vi "LogTimeDataExtract.vi"() -> ()   [LabVIEW 2014]
uses:
  ColumnData.ctl
  <vilib>/Analysis/NI_AALBase.lvlib
panel:
  out "Busy Interval Histogram":T1(graph)
  out "Busy Delay Histogram":T1(graph)
  out "Audible Read Interval Mean":dbl format="%0.4f"
  out "Audible Read Interval Histogram":T1(graph)
  out "Audible Read Start Delay Histogram":T1(graph)
  out "Column Repeat Sample Size":i32
  out "Column Switch Sample Size":i32
  out "Audible Read Start Delay Mean":dbl format="%0.4f"
  out "Column Repeat Command Delay Histogram":T1(graph)
  out "Column Switch Command Delay Histogram":T1(graph)
  out "Column Switch Command Delay Mean":dbl format="%0.4f"
  out "Column Repeat Command Delay Mean":dbl format="%0.4f"
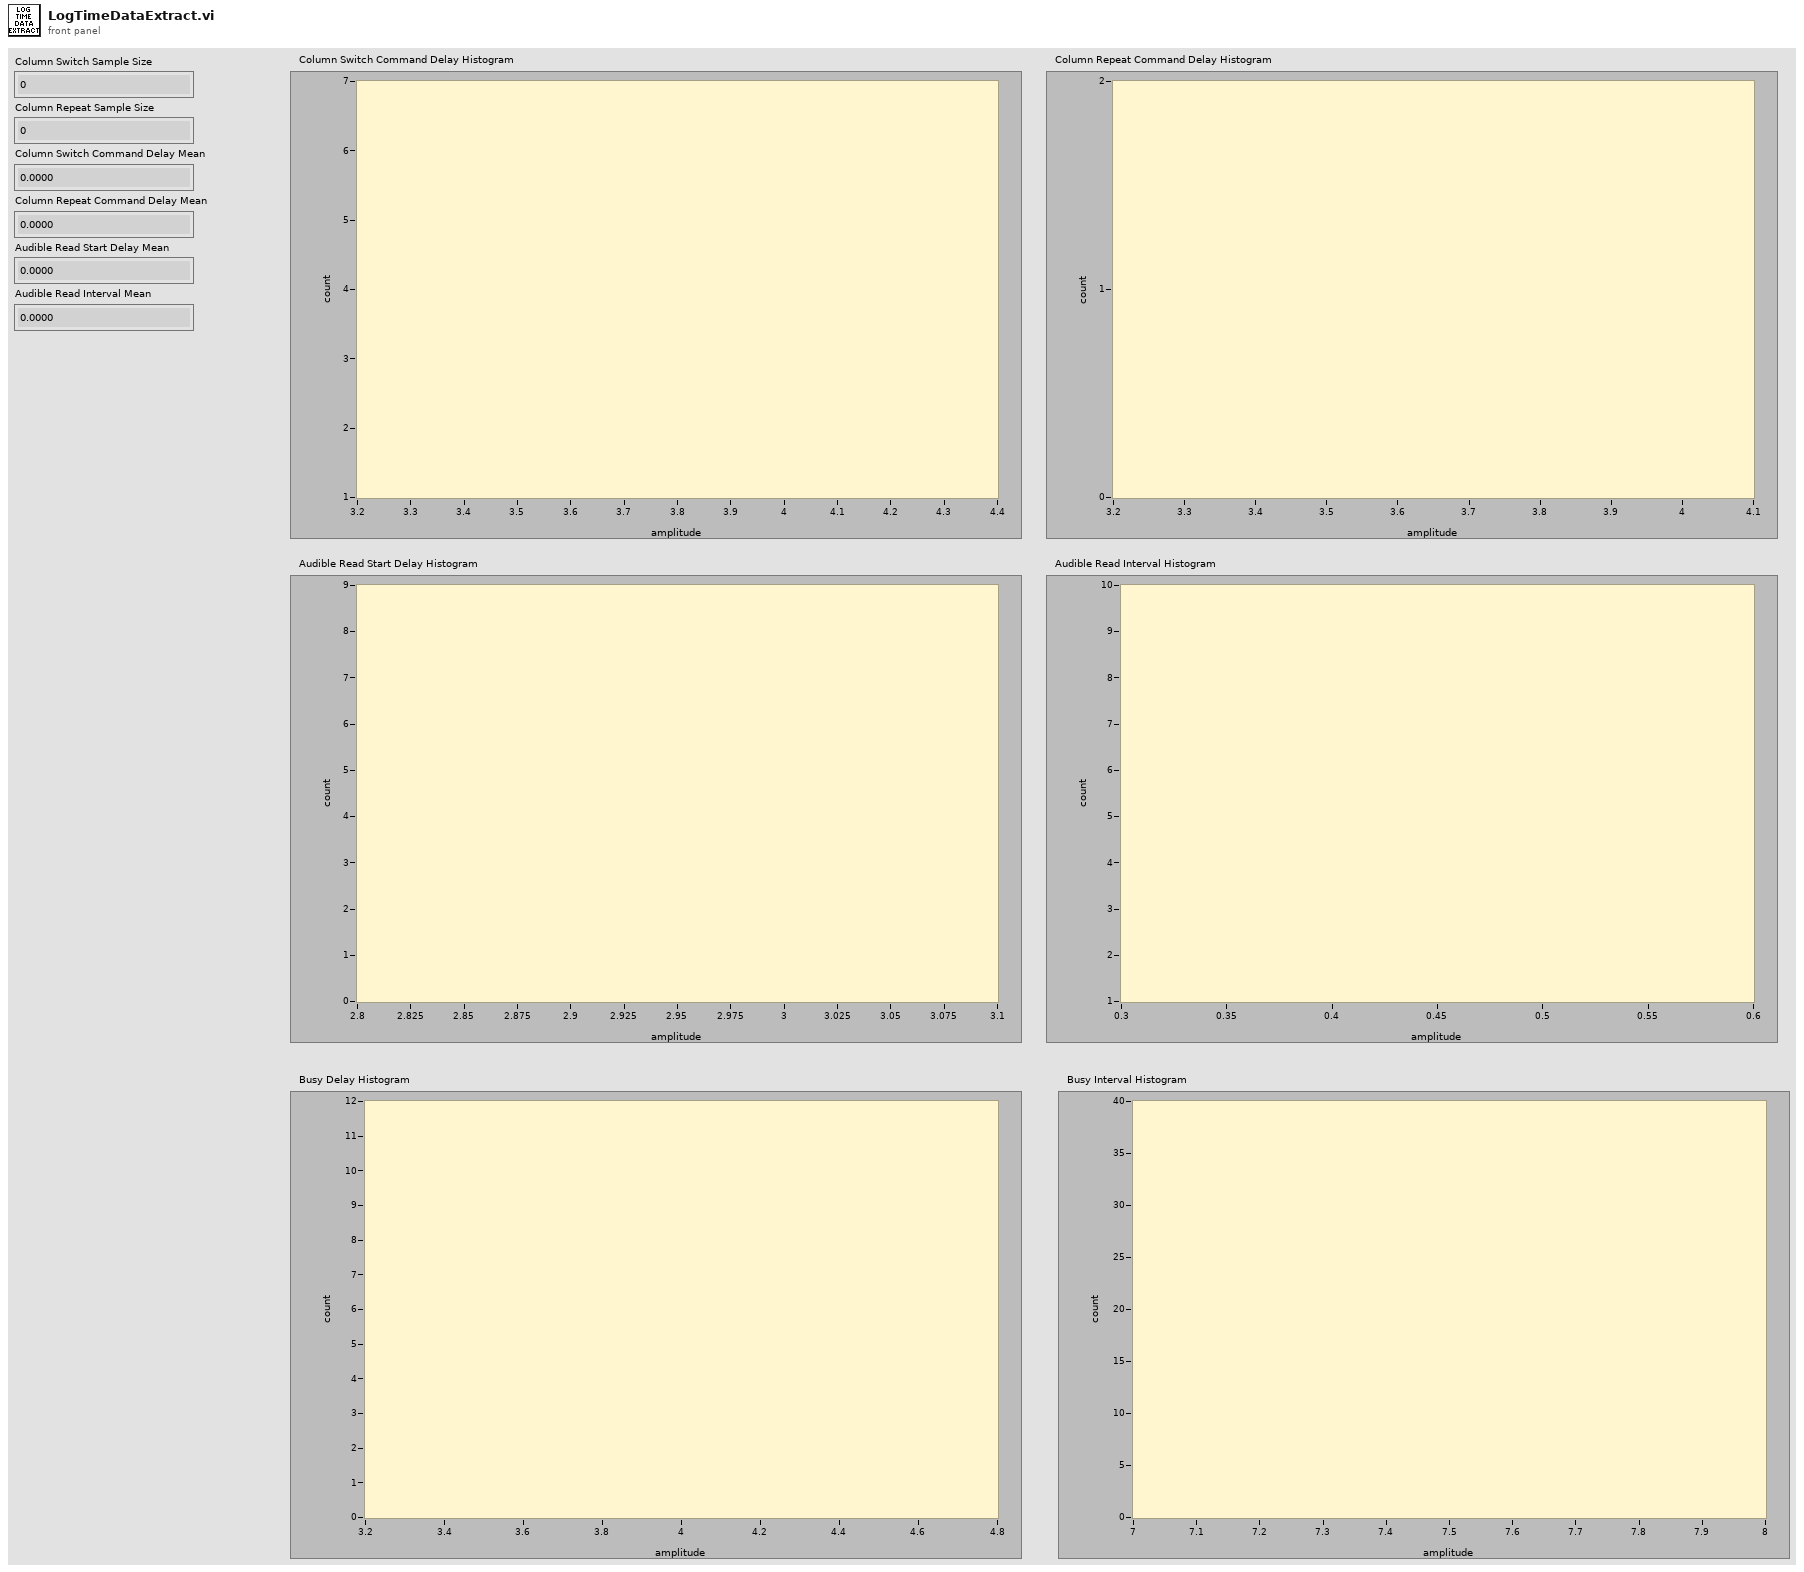
[diagram p1: front panel]
types:
  T1 = cluster{"X Values":dbl[], "Histogram: h(x)":i32[]}
  T2 = typedef "ColumnData.ctl" = cluster{"Col Absorbances":dbl[], "Col Read Times":timestamp[], "Col Read Positions (deg)":dbl[], "Temperature (degC)":dbl, "Active Column":u64, "Previous Column":u64, "Column Read Start Time":timestamp, "Column Busy Start Time":timestamp, "Column Busy Stop Time":timestamp, "Column Mark Read Start Time":timestamp, "Column Mark Read Stop Time":timestamp}
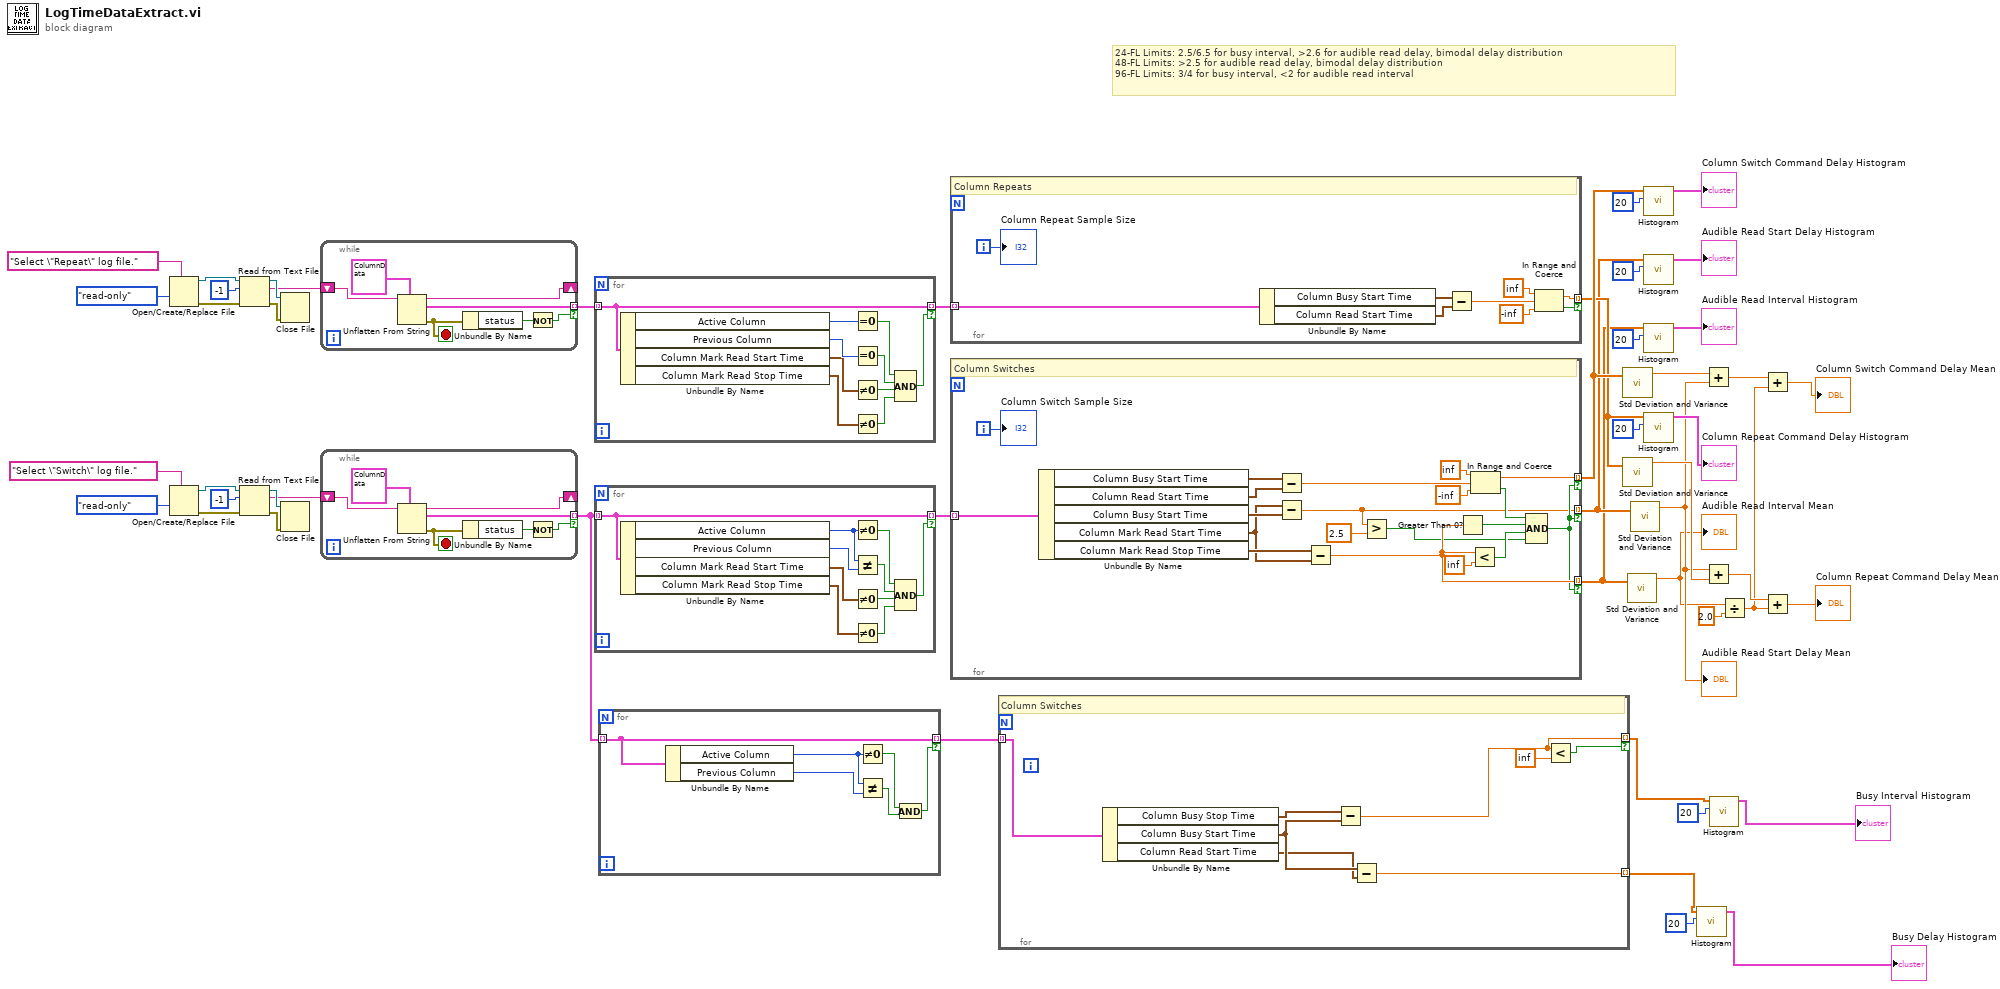
[diagram p0: block diagram]
diagram:
  # "24-FL Limits: 2.5/6.5 for busy interval, >2.6 for audible read delay, bimodal delay distribution\n48-FL Limits: >2.5 for audible read delay, bimodal delay distribution\n96-FL Limits: 3/4 for busy interval, <2 for audible read interval"
  n1 = Open/Create/Replace File(prompt="Select \"Repeat\" log file.", access (0:read/write)=enum16{"read/write", "read-only", "write-only"}."read-only") -> (refnum out=w38:refnum<file>, error out=w35:errorcluster)  [unwired: 4 in, 1 out]
  n2 = Open/Create/Replace File(prompt="Select \"Switch\" log file.", access (0:read/write)=enum16{"read/write", "read-only", "write-only"}."read-only") -> (refnum out=w49:refnum<file>, error out=w46:errorcluster)  [unwired: 4 in, 1 out]
  n3 = Read from Text File(file (use dialog)=w38, count=-1, error in=w35) -> (refnum out=w36:refnum<file>, text=w31:string, error out=w34:errorcluster)  [unwired: 1 in, 1 out]
  n4 = Read from Text File(file (use dialog)=w49, count=-1, error in=w46) -> (refnum out=w47:refnum<file>, text=w30:string, error out=w45:errorcluster)  [unwired: 1 in, 1 out]
  n5 = Close File(refnum=w36, error in=w34) -> ()  [unwired: 2 out]
  n6 = Close File(refnum=w47, error in=w45) -> ()  [unwired: 2 out]
  n7 = while {
    shift-right: [w55] -> _
    shift-left: w31 -> [w56]
    tunnel: [w54] -> w27 mode=indexing if=w50
    stop <- w52 stop-if-true
    n8 = Unflatten From String(type=T2 {"Col Absorbances"=[], "Col Read Times"=[], "Col Read Positions (deg)"=[], "Temperature (degC)"=0.0, "Active Column"=0, "Previous Column"=0, "Column Read Start Time"=timestamp(0 s since 1904-01-01), "Column Busy Start Time"=timestamp(0 s since 1904-01-01), "Column Busy Stop Time"=timestamp(0 s since 1904-01-01), "Column Mark Read Start Time"=timestamp(0 s since 1904-01-01), "Column Mark Read Stop Time"=timestamp(0 s since 1904-01-01)} ("Column Data"), binary string=w56) -> (rest of the binary string=w55:string, value=w54:T2, error out=w52:errorcluster)  [unwired: 3 in]
    n9 = Unbundle By Name(w52) -> ("status"=w51:bool)
    n10 = Not(x=w51) -> (.not. x?=w50:bool)
  }
  n11 = while {
    shift-right: [w62] -> _
    shift-left: w30 -> [w63]
    tunnel: [w61] -> w8 mode=indexing if=w57
    stop <- w59 stop-if-true
    n12 = Unflatten From String(type=T2 {"Col Absorbances"=[], "Col Read Times"=[], "Col Read Positions (deg)"=[], "Temperature (degC)"=0.0, "Active Column"=0, "Previous Column"=0, "Column Read Start Time"=timestamp(0 s since 1904-01-01), "Column Busy Start Time"=timestamp(0 s since 1904-01-01), "Column Busy Stop Time"=timestamp(0 s since 1904-01-01), "Column Mark Read Start Time"=timestamp(0 s since 1904-01-01), "Column Mark Read Stop Time"=timestamp(0 s since 1904-01-01)} ("Column Data"), binary string=w63) -> (rest of the binary string=w62:string, value=w61:T2, error out=w59:errorcluster)  [unwired: 3 in]
    n13 = Unbundle By Name(w59) -> ("status"=w58:bool)
    n14 = Not(x=w58) -> (.not. x?=w57:bool)
  }
  n15 = for {
    tunnel: w27 -> [w69] mode=indexing
    tunnel: [w69] -> w26 mode=indexing if=w68
    n16 = Unbundle By Name(w69) -> ("Active Column"=w73:u64, "Previous Column"=w72:u64, "Column Mark Read Start Time"=w67:timestamp, "Column Mark Read Stop Time"=w64:timestamp)
    n17 = Equal To 0?(x=w73) -> (x = 0?=w70:bool)
    n18 = Equal To 0?(x=w72) -> (x = 0?=w71:bool)
    n19 = Not Equal To 0?(x=w67) -> (x != 0?=w66:bool)
    n20 = Not Equal To 0?(x=w64) -> (x != 0?=w65:bool)
    n21 = Compound Arithmetic op=AND(w70, w71, w66, w65) -> (w68:bool)
  }
  n22 = for {
    tunnel: w8 -> [w83] mode=indexing
    tunnel: [w83] -> w9 mode=indexing if=w78
    n23 = Unbundle By Name(w83) -> ("Active Column"=w82:u64, "Previous Column"=w81:u64, "Column Mark Read Start Time"=w77:timestamp, "Column Mark Read Stop Time"=w75:timestamp)
    n24 = Not Equal To 0?(x=w82) -> (x != 0?=w80:bool)
    n25 = Not Equal?(x=w82, y=w81) -> (x != y?=w79:bool)
    n26 = Not Equal To 0?(x=w77) -> (x != 0?=w76:bool)
    n27 = Not Equal To 0?(x=w75) -> (x != 0?=w74:bool)
    n28 = Compound Arithmetic op=AND(w80, w79, w76, w74) -> (w78:bool)
  }
  n29 = for {
    tunnel: w8 -> [w89] mode=indexing
    tunnel: [w89] -> w7 mode=indexing if=w84
    n30 = Unbundle By Name(w89) -> ("Active Column"=w88:u64, "Previous Column"=w87:u64)
    n31 = Not Equal To 0?(x=w88) -> (x != 0?=w86:bool)
    n32 = Not Equal?(x=w88, y=w87) -> (x != y?=w85:bool)
    n33 = Compound Arithmetic op=AND(w86, w85) -> (w84:bool)
  }
  n34 = for {
    tunnel: w26 -> [w98] mode=indexing
    tunnel: [w93] -> w32 mode=indexing if=w92
    i -> [w95]
    # "Column Repeats"
    n35 = Unbundle By Name(w98) -> ("Column Busy Start Time"=w97:timestamp, "Column Read Start Time"=w96:timestamp)
    n36 = Subtract(x=w97, y=w96) -> (x-y=w94:dbl)
    n37 = In Range and Coerce(upper limit=inf, x=w94, lower limit=-inf) -> (coerced(x)=w93:dbl, In Range?=w92:bool)
    "Column Repeat Sample Size" <- w95
  }
  n38 = for {
    tunnel: w9 -> [w118] mode=indexing
    tunnel: [w115] -> w39 mode=indexing if=w104
    tunnel: [w103] -> w23 mode=indexing if=w104
    tunnel: [w112] -> w21 mode=indexing if=w104
    i -> [w116]
    # "Column Switches"
    n39 = Unbundle By Name(w118) -> ("Column Busy Start Time"=w117:timestamp, "Column Read Start Time"=w108:timestamp, "Column Busy Start Time"=w107:timestamp, "Column Mark Read Start Time"=w105:timestamp, "Column Mark Read Stop Time"=w106:timestamp)
    n40 = Subtract(x=w117, y=w108) -> (x-y=w109:dbl)
    n41 = Subtract(x=w105, y=w107) -> (x-y=w103:dbl)
    n42 = Subtract(x=w106, y=w105) -> (x-y=w112:dbl)
    n43 = Greater?(x=w103, y=2.5) -> (0:w102:bool)
    n44 = Greater Than 0?(x=w112) -> (x > 0?=w113:bool)
    n45 = Less?(x=w112, y=inf) -> (x < y?=w110:bool)
    n46 = In Range and Coerce(upper limit=inf, x=w109, lower limit=-inf) -> (coerced(x)=w115:dbl, In Range?=w114:bool)
    n47 = Compound Arithmetic op=AND(w114, w113, w110, w102) -> (w104:bool)
    "Column Switch Sample Size" <- w116
  }
  n48 = for {
    tunnel: w7 -> [w126] mode=indexing
    tunnel: [w122] -> w4 mode=indexing
    tunnel: [w120] -> w1 mode=indexing if=w119
    # "Column Switches"
    n49 = Unbundle By Name(w126) -> ("Column Busy Stop Time"=w125:timestamp, "Column Busy Start Time"=w124:timestamp, "Column Read Start Time"=w123:timestamp)
    n50 = Subtract(x=w125, y=w124) -> (x-y=w120:dbl)
    n51 = Subtract(x=w124, y=w123) -> (x-y=w122:dbl)
    n52 = Less?(x=w120, y=inf) -> (x < y?=w119:bool)
  }
  n53 = call <vilib>:"Std Deviation and Variance.vi"("X"=w39) -> ("mean"=w19:dbl)  [unwired: 1 in, 2 out]
  n54 = call <vilib>:"Std Deviation and Variance.vi"("X"=w32) -> ("mean"=w18:dbl)  [unwired: 1 in, 2 out]
  n55 = call <vilib>:"Std Deviation and Variance.vi"("X"=w21) -> ("mean"=w16:dbl)  [unwired: 1 in, 2 out]
  "Audible Read Interval Mean" <- w16
  n56 = call <vilib>:"Std Deviation and Variance.vi"("X"=w23) -> ("mean"=w17:dbl)  [unwired: 1 in, 2 out]
  "Audible Read Start Delay Mean" <- w17
  n57 = call <vilib>:"Histogram.vi"("intervals"=20, "X"=w39) -> ("Histogram Graph"=→"Column Switch Command Delay Histogram":T1)  [unwired: 6 in, 3 out]
  n58 = call <vilib>:"Histogram.vi"("intervals"=20, "X"=w23) -> ("Histogram Graph"=→"Audible Read Start Delay Histogram":T1)  [unwired: 6 in, 3 out]
  n59 = call <vilib>:"Histogram.vi"("intervals"=20, "X"=w21) -> ("Histogram Graph"=→"Audible Read Interval Histogram":T1)  [unwired: 6 in, 3 out]
  n60 = call <vilib>:"Histogram.vi"("intervals"=20, "X"=w32) -> ("Histogram Graph"=→"Column Repeat Command Delay Histogram":T1)  [unwired: 6 in, 3 out]
  n61 = call <vilib>:"Histogram.vi"("intervals"=20, "X"=w4) -> ("Histogram Graph"=→"Busy Delay Histogram":T1)  [unwired: 6 in, 3 out]
  n62 = Add(x=w19, y=w17) -> (x+y=w11:dbl)
  n63 = Add(x=w17, y=w18) -> (x+y=w14:dbl)
  n64 = call <vilib>:"Histogram.vi"("intervals"=20, "X"=w1) -> ("Histogram Graph"=→"Busy Interval Histogram":T1)  [unwired: 6 in, 3 out]
  n65 = Divide(x=w16, y=2.0) -> (x/y=w10:dbl)
  n66 = Add(x=w11, y=w10) -> (x+y=→"Column Switch Command Delay Mean":dbl)
  n67 = Add(x=w14, y=w10) -> (x+y=→"Column Repeat Command Delay Mean":dbl)
